vi "Static Write.vi"(8 "error in (no error)":errorcluster, 10 "Array":string[](array[string]), 11 "Abs_String in":refnum<class "Abs_String 1D.lvclass">) -> (0 "error out":errorcluster, 3 "Abs_String out":refnum<class "Abs_String 1D.lvclass">)   [LabVIEW 2021, in "Abs_String 1D.lvclass"]
uses:
  Abs_String 1D.lvclass
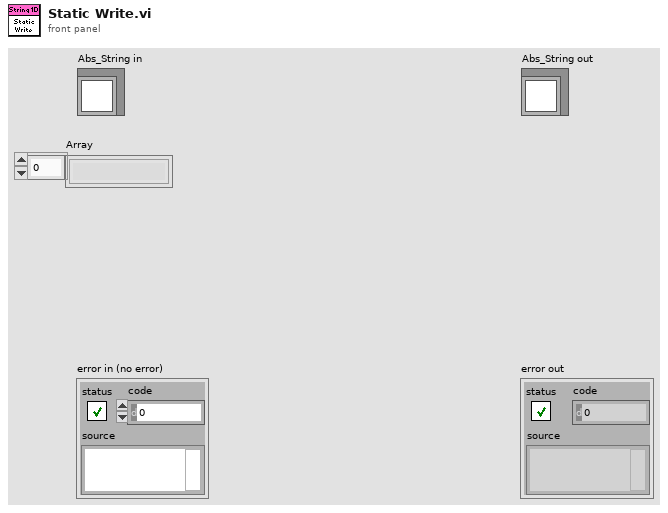
[diagram p1: front panel]
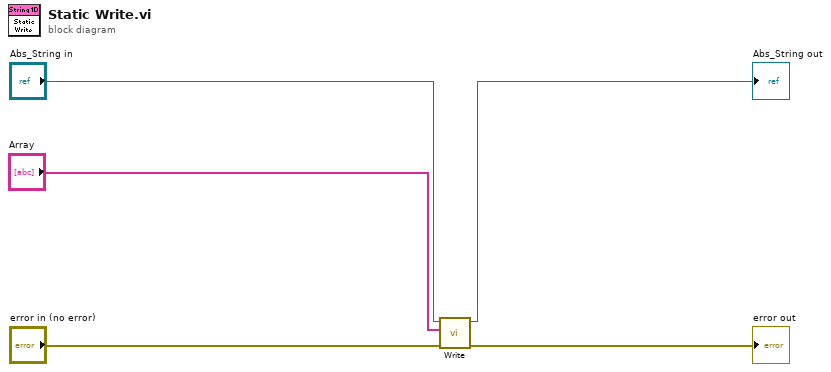
[diagram p0: block diagram]
diagram:
  n1 = call-dynamic "Write.vi"("error in (no error)"="error in (no error)", "Array"="Array", "Abs_String in"="Abs_String in") -> ("error out"=→"error out":errorcluster, "Abs_String out"=→"Abs_String out":refnum<class "Abs_String 1D.lvclass">)  [unwired: 7 in]
